vi "DSF.Shared.Configuration.Transfer.Load from Disk.vi"(8 "error in (no error)":errorcluster, 10 "class path":path, 11 "Transfer Configuration in":refnum<class "DSF.Shared.Configuration.Transfer.lvclass">) -> (0 "error out":errorcluster, 3 "Transfer Configuration out":refnum<class "DSF.Shared.Configuration.Transfer.lvclass">)   [LabVIEW 2016, in "DSF.Shared.lvlib" / "DSF.Shared.Configuration.Transfer.lvclass"]
uses:
  DSF.Shared.Configuration.Transfer.lvclass
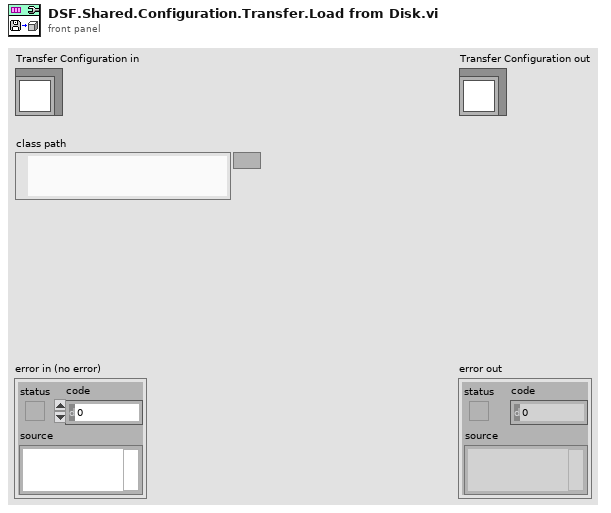
[diagram p1: front panel]
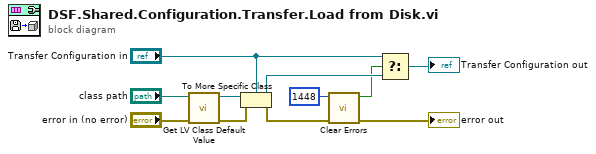
[diagram p0: block diagram]
diagram:
  n1 = call <vilib>:"Get LV Class Default Value.vi"("error in (no error)"="error in (no error)", "class path"="class path") -> ("error out"=w9:errorcluster, "object"=w10:refnum<class>)  [unwired: 8 in]
  n2 = To More Specific Class(target class="Transfer Configuration in", reference=w10, error in=w9) -> (specific class reference=w7:refnum<class "DSF.Shared.Configuration.Transfer.lvclass">, error out=w8:errorcluster)
  n3 = call <vilib>:"Clear Errors.vi"("error in (no error)"=w8, "specific error code to clear (0: all)"=1448) -> ("error out"=→"error out":errorcluster, "specific error cleared?"=w6:bool)  [unwired: 4 in]
  n4 = Select(t="Transfer Configuration in", s=w6, f=w7) -> (s? t:f=→"Transfer Configuration out":refnum<class "DSF.Shared.Configuration.Transfer.lvclass">)
